vi "_Test_Demo_Checkbox.vi"() -> ()   [LabVIEW 2023]
uses:
  DSLV_Tree/DSLV_Tree.lvlib
panel:
  in  "Tri-State?":bool=TRUE
  out "Seted Tags":T1(array[cluster])
  out "error out":errorcluster
  in  "Tree":string(tree)
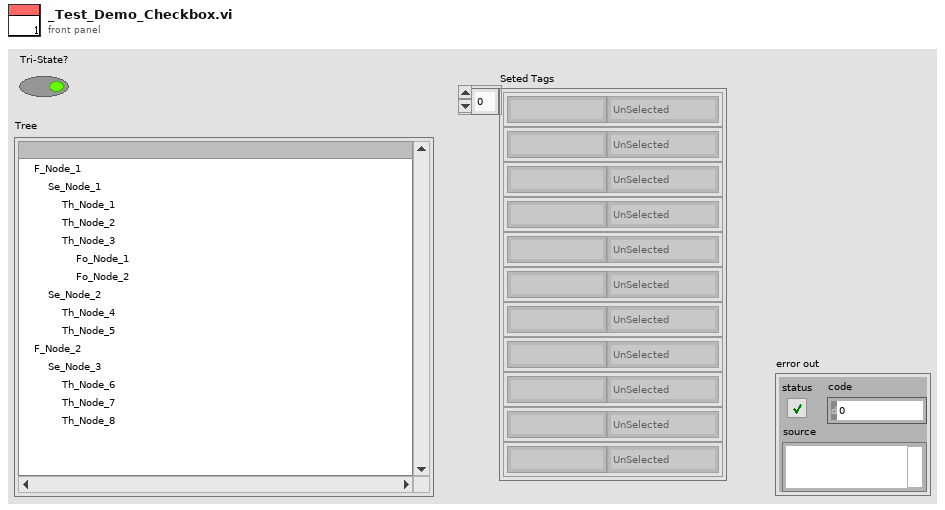
[diagram p1: front panel]
types:
  T1 = cluster{"Tag":string, "Selected?":enum16{"UnSelected", "Selected", "PartSelected"}}[]
  T2 = typedef "LVPoint32TypeDef.ctl" = cluster{"Horizontal":i32, "Vertical":i32}
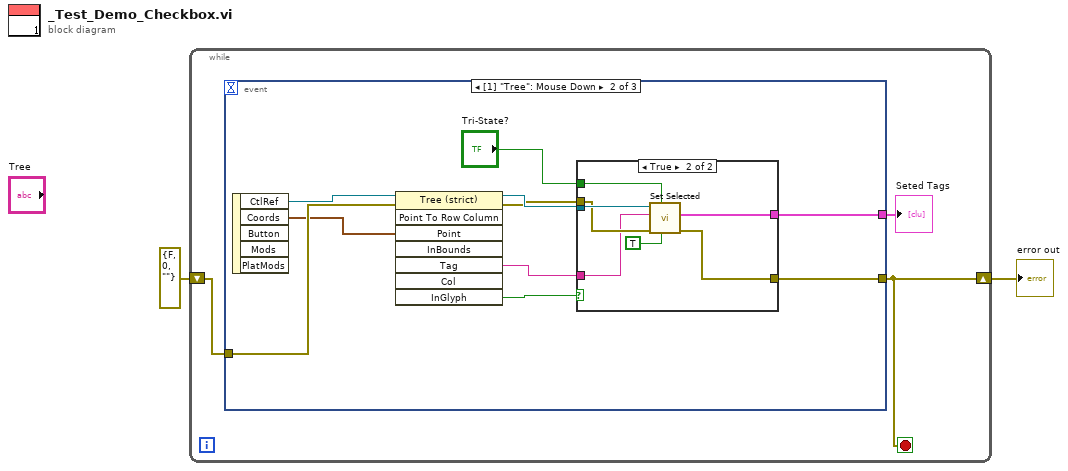
[diagram p0: block diagram]
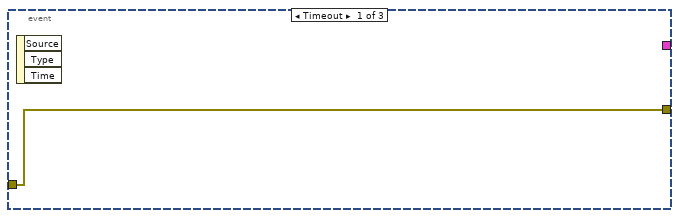
[diagram p2: hidden frame]
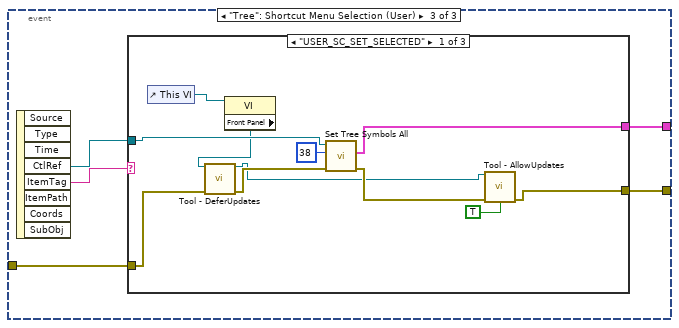
[diagram p4: hidden frame]
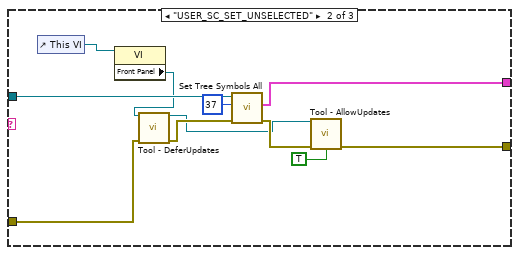
[diagram p5: hidden frame]
diagram:
  n1 = while {
    shift-right: [w4] -> w2
    shift-left: errorcluster {"status"=FALSE, "code"=0, "source"=""} ("error out") -> [w5]
    stop <- w4 stop-if-true
    n2 = event shown="[1] \"Tree\": Mouse Down" {
      selector: _ -> [_ _ _]
      dyn-events: _ -> [_ _ _]
      timeout: _ -> [_ _ _]
      tunnel: [w6 w16 w27] -> w4
      tunnel: w5 -> [w6 w12 w26]
      tunnel: [_ w15 w25] -> w3
      event Timeout {
        n3 = event-data() -> ()  [unwired: 1 in, 3 out]
      }
      event "Tree": Mouse Down {
        n4 = event-data() -> ("CtlRef"=w14:refnum<vi>, "Coords"=w10:T2)  [unwired: 1 in, 3 out]
        n5 = invoke on="Invoke Node" class="Tree (strict)" method="Point To Row Column"(reference=w14, error in=w12, "Point"=w10) -> (reference out=w13:refnum<vi>, error out=w11:errorcluster, "Tag"=w8:string, "InGlyph"=w9:bool)  [unwired: 5 in, 4 out]
        n6 = case shown="True" w9 {
          tunnel: [w17 w24] -> w16
          tunnel: [_ w23] -> w15
          tunnel: w13 -> [_ w22]
          tunnel: w11 -> [w17 w21]
          tunnel: w8 -> [_ w19]
          tunnel: "Tri-State?" -> [_ w18]
          frame False {
          }
          frame True {
            n7 = call "Set Selected.vi"("Get All Children?"=TRUE, "Tri-State?"=w18, "error in (no error)"=w21, "Tag"=w19, "Tree Reference"=w22) -> ("error out"=w24:errorcluster, "Seted Tags"=w23:T1)  [unwired: 4 in, 1 out]
          }
        }
      }
      event "Tree": Shortcut Menu Selection (User) {
        n8 = event-data() -> ("CtlRef"=w28:refnum<vi>, "ItemTag"=w29:string)  [unwired: 1 in, 6 out]
        n9 = case shown="\"USER_SC_SET_SELECTED\"" w29 {
          tunnel: w28 -> [w39 w51 _]
          tunnel: [w32 w43 w52] -> w27
          tunnel: w26 -> [w31 w42 w52]
          tunnel: [w30 w41 _] -> w25
          frame "USER_SC_SET_SELECTED" {
            n10 = control-ref of="This VI"() -> (w38:refnum<vi>)
            n11 = property class="VI"(reference=w38) -> ("Front Panel"=w37:refnum<vi>)  [unwired: 1 in, 2 out]
            n12 = call "Tool - DeferUpdates.vi"("Panel Ref In"=w37, "error in (no error)"=w31) -> ("Panel Ref Out"=w34:refnum<vi>, "error out"=w36:errorcluster)  [unwired: 12 in]
            n13 = call "Set Tree Symbols All.vi"("error in (no error)"=w36, "symbol"=38, "Tree Refnum"=w39) -> ("error out"=w35:errorcluster, "Seted Tags"=w30:T1)  [unwired: 6 in, 1 out]
            n14 = call "Tool - AllowUpdates.vi"("Panel ref in"=w34, "error in (no error)"=w35, "Clear Ref? (F)"=TRUE) -> ("error out"=w32:errorcluster)  [unwired: 11 in, 1 out]
          }
          frame "USER_SC_SET_UNSELECTED" {
            n15 = control-ref of="This VI"() -> (w49:refnum<vi>)
            n16 = property class="VI"(reference=w49) -> ("Front Panel"=w46:refnum<vi>)  [unwired: 1 in, 2 out]
            n17 = call "Tool - DeferUpdates.vi"("Panel Ref In"=w46, "error in (no error)"=w42) -> ("Panel Ref Out"=w45:refnum<vi>, "error out"=w48:errorcluster)  [unwired: 12 in]
            n18 = call "Set Tree Symbols All.vi"("error in (no error)"=w48, "symbol"=37, "Tree Refnum"=w51) -> ("error out"=w47:errorcluster, "Seted Tags"=w41:T1)  [unwired: 6 in, 1 out]
            n19 = call "Tool - AllowUpdates.vi"("Panel ref in"=w45, "error in (no error)"=w47, "Clear Ref? (F)"=TRUE) -> ("error out"=w43:errorcluster)  [unwired: 11 in, 1 out]
          }
          frame Default {
          }
        }
      }
    }
    "Seted Tags" <- w3
  }
  "error out" <- w2
